vi "Create_Waveforms.vi"(8 "error in":errorcluster caption="entrée d'erreur", 9 "Timings (sleep, expo, readout) _s":dbl[](array[numeric])=[0.025, 0.1, 0.02], 10 "sample_rate_Hz":dbl=100000.0, 11 "Trajectories":cluster{dbl[], dbl[]}(graph)={[0.0, 0.03117691453623979, 0.036, 0.0, -0.072, -0.15588457268119893, -0.21599999999999997, -0.21823840175367853, -0.144, 0.0, 0.18, 0.34294605989863763, 0.43199999999999994, 0.43199999999999994, 0.4284998350783742, 0.3677013326971094, 0.25199999999999995, 0.0916862378081392, -0.09585379407214553, -0.288, -0.45962666587138673, -0.5863681953704067, -0.6479999999999999, -0.6314734411681304, -0.5331669324108087, -0.36, -0.12919424418419617, 0.13336180044820248, 0.39599999999999996, 0.6250922655850859, 0.789341801460163, 0.8639999999999999, 0.8639999999999999, 0.8519465787869581, 0.7794228634059946, 0.6491240251292506, 0.4679999999999999, 0.24691336902780475, 0.0, -0.2562308546514955, -0.5039999999999999, -0.7254915574973977, -0.9041305215509537, -1.0258132275189904, -1.0799999999999998, -1.060586557265397, -0.9664843506234334, -0.8018590898655449, -0.576, -0.30281828276994927, 0.0, 0.31213576839364, 0.6119999999999999, 0.878226622233692, 1.0911920087683924, 1.2344532059974291, 1.2959999999999998, 1.2959999999999998, 1.2881285409399679, 1.240394259437399, 1.153545837840872, 1.0295637315519064, 0.8716199987349471, 0.6839999999999999, 0.4719877977894228, 0.241718263312367, 0.0, -0.24588581957637334, -0.4884047646690548, -0.7199999999999999, -0.9333276092648548, -1.1214890647261837, -1.2782534959858312, -1.3982626197294314, -1.4772116295183118, -1.5119999999999998, -1.5008470155906048, -1.4433678655271551, -1.3406073250583108, -1.1950293312656055, -1.0104621224272397, -0.7919999999999999, -0.5458641487477672, -0.27922626968842396, 0.0, 0.28339382595243023, 0.5622811156273992, 0.8279999999999998, 1.0721697329571473, 1.2869546644398828, 1.46531498320327, 1.6012362258191877, 1.6899301041689487, 1.7279999999999998, 1.7279999999999998, 1.7274016064910866, 1.7135654902412418, 1.686506492700713, 1.6463414716169114, 1.5932890896104304, 1.5276688122757496, 1.4498991183915153, 1.3604949309793049, 1.2600642840744276, 1.149304246119532, 1.0289961268137766, 0.8999999999999999, 0.7632485807037032, 0.6197404997061117, 0.47053302399638264, 0.3167342760644809, 0.15949500922821444, 0.0, -0.1605408781411863, -0.32090183232848724, -0.47985050962007336, -0.6361574665857437, -0.788605676408145, -0.9359999999999998, -1.0771765474672643, -1.2110118566494397, -1.3364318164425746, -1.4524202641535822, -1.5580271882376622, -1.6523764704207087, -1.7346731043881478, -1.804209831908944, -1.8603731414327453, -1.9026485788195857, -1.9306253249018026, -1.9439999999999997, -1.9425796612789035, -1.9262839648918786, -1.8951464711791517, -1.8493150777066676, -1.7890515716103468, -1.7147302994931881, -1.6268359599579376, -1.525960530693004, -1.412799348810722, -1.2881463698118243, -1.1528886370656024, -1.0079999999999998, -0.8545341252396942, -0.693616850664456, -0.5264379377385271, -0.3542422824405378, -0.1783206496617086, 0.0, 0.1793665185746805, 0.3584098387045441, 0.5357554233622179, 0.7100338175440881, 0.8798912209441362, 1.0439999999999998, 1.2010690577190903, 1.3498539803417322, 1.4891668811788692, 1.6178858638672813, 1.7349640298040845, 1.8394379576381472, 1.9304355863880642, 2.0071834379987, 2.069013119911184, 2.1153670534702225, 2.1458033796896196, 2.1599999999999997], [0.0, 0.023999474994257686, 0.0831366200900662, 0.1439968499655461, 0.1662732401801324, 0.11999737497128843, 0.0, -0.1679963249598038, -0.3325464803602648, -0.4319905498966383, -0.41568310045033097, -0.26399422493683455, 0.0, 0.0, 0.207943698224346, 0.41137507107442045, 0.5819563406304633, 0.6932894919153157, 0.7248026506387393, 0.6650929607205296, 0.5142188388430255, 0.2845545344122629, 0.0, -0.30644334475166773, -0.5964938530579097, -0.8313662009006619, -0.976907920426127, -1.0084210791495503, -0.9145028209907282, -0.6993376208265146, -0.3830541809395847, 0.0, 0.0, 0.30436453884780434, 0.5999868748564421, 0.865479767181186, 1.0807760611708606, 1.2286307738596058, 1.295971649689915, 1.2749941992882703, 1.1639126812609266, 0.9673009162613255, 0.6959847748334728, 0.3664797508575603, 0.0, -0.3789027932595115, -0.7439837248219882, -1.069122065341465, -1.3301859214410592, -1.506811326431592, -1.5839653496210069, -1.5531747518602566, -1.413322541531125, -1.1709432144216045, -0.8399816247990189, -0.44101800526926743, 0.0, 0.0, 0.3028357971006895, 0.6019422843336332, 0.8879805747875343, 1.1518501990083772, 1.3849780557700053, 1.5795957817112578, 1.7289965992043907, 1.8277632059585598, 1.8719590495520995, 1.8592763646819834, 1.78913561135063, 1.6627324018013239, 1.483029599541333, 1.2546939667769823, 0.983978474764565, 0.67855312052155, 0.3472887581429925, 0.0, -0.3528453782732804, -0.7004419308609549, -1.0319774247530804, -1.3369689809918666, -1.605594029255493, -1.8290056419814564, -1.999622153862469, -2.111381634469371, -2.159952749483191, -2.1428947931927937, -2.0597611660087085, -1.9121422620715223, -1.7036455730268207, -1.4398127487604715, -1.1279753247301112, -0.7770527670488717, -0.3972983393155834, 0.0, 0.0, 0.2014996692826837, 0.4028549594458713, 0.602517556494633, 0.7989415773882768, 0.9905955355318105, 1.1759742747186266, 1.3536107785810658, 1.5220877629753555, 1.6800489598223023, 1.8262100027409804, 1.959368827339736, 2.0784155022516546, 2.1823414108994057, 2.270247708520548, 2.3413529841475507, 2.395000062980182, 2.430661890870268, 2.447946449414284, 2.446600657367777, 2.4265132217036056, 2.387716409576215, 2.3303867206667874, 2.2548444478063625, 2.161552122341721, 2.0511118493556433, 1.924261546512308, 1.7818701089024418, 1.6249315307439607, 1.4545580230854165, 1.2719721746956572, 1.0784982110397527, 0.8755524135761936, 0.6646327685043889, 0.44730792048817436, 0.2252055127277053, 0.0, -0.22659997410682423, -0.45286454061846226, -0.6770558109063401, -0.8974412239155984, -1.1123069323889614, -1.3199711246841725, -1.5187971786790941, -1.707206544958845, -1.8836912579825815, -2.046825976226468, -2.1952794553806405, -2.3278253625218532, -2.4433523437644507, -2.540873263178626, -2.619533536719537, -2.6786184914909925, -2.7175596878254473, -2.735940149345376, -2.733498454322957, -2.710131650214416, -2.6658969621482016, -2.6010122753248655, -2.5158553806714075, -2.4109619826119193, -2.287022477396548, -2.1448775199977956, -1.9855124070627208, -1.8100503127274499, -1.6197444231834448, -1.4159690246612033, -1.2002096078969036, -0.9740520601035154, -0.7391710229160963, -0.4973175016607652, -0.2503058175518459, 0.0]}) -> (0 "error out":errorcluster caption="sortie d'erreur", 1 "Dimension":i32, 2 "DO WF":waveform(dbl)(graph), 3 "AO WF":waveform(dbl)[](graph)=[{"t0"=timestamp(0 s since 1904-01-01), "dt"=inf, "Y"=[]}, {"t0"=timestamp(0 s since 1904-01-01), "dt"=inf, "Y"=[]}])   [LabVIEW 2025]
uses:
  Controls/TypeDef_FGV.ctl
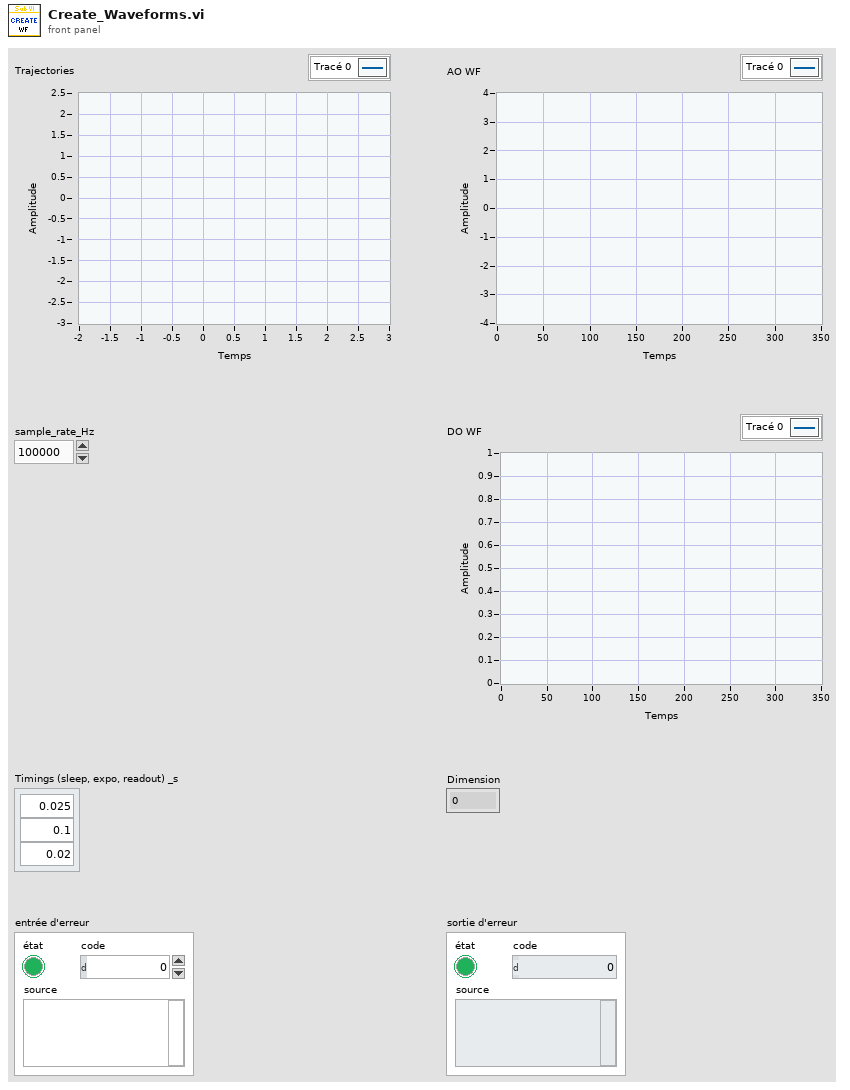
[diagram p1: front panel]
types:
  T1 = typedef "TypeDef_FGV.ctl" = enum16{"Initialize", "Write", "Read"}
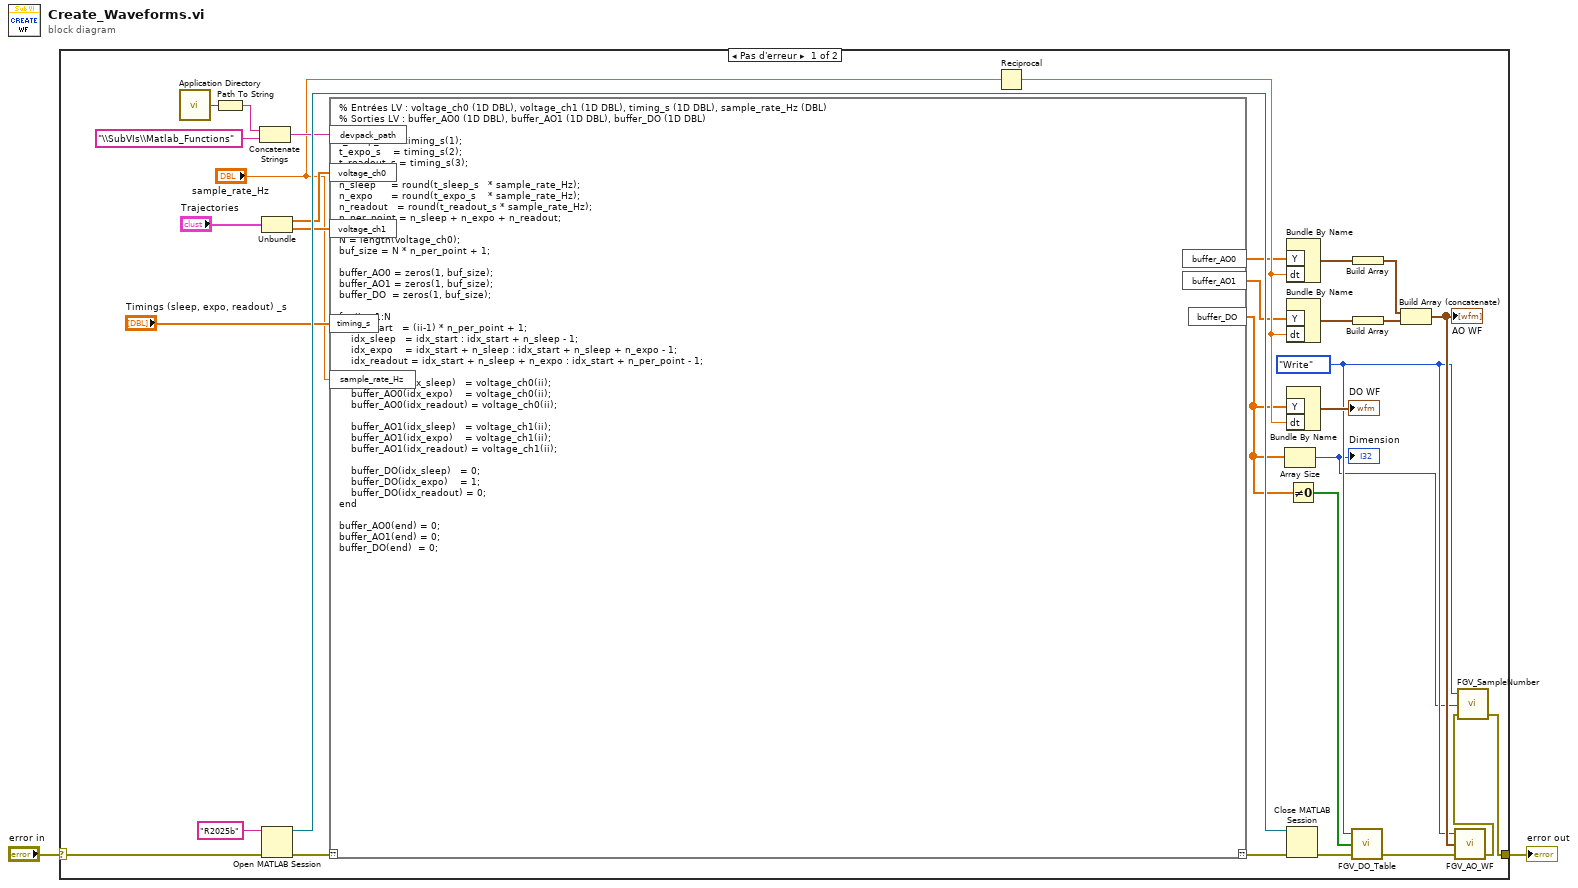
[diagram p0: block diagram]
diagram:
  n1 = case shown="Pas d'erreur" "error in" {
    selector: "error in" -> [w32 w34]
    tunnel: [w5 w34] -> w1
    frame No Error {
      w4 = TypeDef_FGV."Write" ("Action 2")
      n2 = call <vilib>:"Application Directory.vi"() -> ("Application Directory"=w28:path)
      n3 = Path To String(path=w28) -> (string=w29:string)
      n4 = Concatenate Strings(w29, "\\SubVIs\\Matlab_Functions" ("chaîne")) -> (w21:string)
      n5 = Unbundle("Trajectories") -> (w25:dbl[], w23:dbl[])
      n6 = Open MATLAB Session(0:"R2025b" ("nom de version"), 3:w32) -> (8:w33:refnum<k37>, 11:w27:errorcluster)
      n7 = script code="% Entrées LV : voltage_ch0 (1D DBL), voltage_ch1 (1D DBL), timing_s (1D DBL), sample_rate_Hz (DBL)\n% Sorties LV : buffer_AO0 (1D DBL), buffer_AO1 (1D DBL), buffer_DO (1D DBL)\n\nt_sleep_s   = timing_s(1);\nt_expo_s    = timing_s(2);\nt_readout_s = timing_s(3);\n\nn_sleep     = round(t_sleep_s   * sample_rate_Hz);\nn_expo      = round(t_expo_s    * sample_rate_Hz);\nn_readout   = round(t_readout_s * sample_rate_Hz);\nn_per_point = n_sleep + n_expo + n_readout;\n\nN = length(voltage_ch0);\nbuf_size = N * n_per_point + 1;\n\nbuffer_AO0 = zeros(1, buf_size);\nbuffer_AO1 = zeros(1, buf_size);\nbuffer_DO  = zeros(1, buf_size);\n\nfor ii = 1:N\n    idx_start   = (ii-1) * n_per_point + 1;\n    idx_sleep   = idx_start : idx_start + n_sleep - 1;\n    idx_expo    = idx_start + n_sleep : idx_start + n_sleep + n_expo - 1;\n    idx_readout = idx_start + n_sleep + n_expo : idx_start + n_per_point - 1;\n\n    buffer_AO0(idx_sleep)   = voltage_ch0(ii);\n    buffer_AO0(idx_expo)    = voltage_ch0(ii);\n    buffer_AO0(idx_readout) = voltage_ch0(ii);\n\n    buffer_AO1(idx_sleep)   = voltage_ch1(ii);\n    buffer_AO1(idx_expo)    = voltage_ch1(ii);\n    buffer_AO1(idx_readout) = voltage_ch1(ii);\n\n    buffer_DO(idx_sleep)   = 0;\n    buffer_DO(idx_expo)    = 1;\n    buffer_DO(idx_readout) = 0;\nend\n\nbuffer_AO0(end) = 0;\nbuffer_AO1(end) = 0;\nbuffer_DO(end)  = 0;"("??"=w27, "voltage_ch0"=w25, "voltage_ch1"=w23, "sample_rate_Hz"="sample_rate_Hz", "timing_s"="Timings (sleep, expo, readout) _s", "devpack_path"=w21) -> ("??"=w26:errorcluster, "buffer_AO0"=w12:dbl[], "buffer_AO1"=w11:dbl[], "buffer_DO"=w8:dbl[])
      n8 = Reciprocal(x="sample_rate_Hz") -> (1/x=w15:dbl)
      n9 = Array Size(array=w8) -> (size(s)=w3:i32)
      "Dimension" <- w3
      n10 = Bundle By Name("Y"=w12, "dt"=w15) -> (w14:waveform(dbl))  [unwired: 1 in]
      n11 = Bundle By Name("Y"=w11, "dt"=w15) -> (w13:waveform(dbl))  [unwired: 1 in]
      n12 = Bundle By Name("Y"=w8, "dt"=w15) -> (→"DO WF":waveform(dbl))  [unwired: 1 in]
      n13 = Close MATLAB Session(0:w33, 3:w26) -> (11:w20:errorcluster)
      n14 = Not Equal To 0?(x=w8) -> (x != 0?=w7:bool[])
      n15 = call "FGV_DO_Table.vi"("error in"=w20, "DO table"=w7, "Action"=w4) -> ("error out"=w19:errorcluster)  [unwired: 1 in, 1 out]
      n16 = Build Array(w14) -> (w17:waveform(dbl)[])
      n17 = Build Array(w13) -> (w16:waveform(dbl)[])
      n18 = Build Array (concatenate)(w17, w16) -> (w9:waveform(dbl)[])
      "AO WF" <- w9
      n19 = call "FGV_AO_WF.vi"("error in 2"=w19, "AO WF 3"=w9, "Action 2"=w4) -> ("error out 2"=w6:errorcluster)  [unwired: 1 in, 1 out]
      n20 = call "FGV_SampleNumber.vi"("error in"=w6, "Sample number"=w3, "Action"=w4) -> ("error out"=w5:errorcluster)  [unwired: 1 in, 1 out]
    }
    frame Error {
    }
  }
  "error out" <- w1
